vi "Read Registration Refnum.vi"(6 "Event Type":T1, 7 "TreeControlEventHandler":refnum<class "TreeControlEventHandler.lvclass">) -> (1 "TreeControl Refnum":refnum<vi>)   [LabVIEW 2020, in "MVA Framework.lvlib" / "ActorEvents.lvlib" / "TreeControlEventHandler.lvclass"]
doc: "读取注册树形引用"
uses:
  TreeControlEventHandler.lvclass
  <vilib>/event_ctls.llb/lveventtype.ctl
  IEventHandler/IEventHandler.lvclass/IEventHandler.ctl
  TreeControlEventHandler.lvclass/TreeControlEventHandler.ctl
  IEventHandler/IEventHandler.lvclass
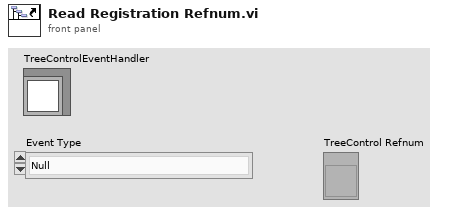
[diagram p1: front panel]
types:
  T1 = typedef "lveventtype.ctl" = enum32{"Null", "Timeout", "Annotation Menu Selection", "Annotation Menu Selection?", "App Instance Close", "App Instance Close?", "Autoscale Range Change", "Bookmark Info Change", "Cell Edit", "Cell Edit?", "Cursor Grab", "Cursor Grab?", "Cursor Menu Selection", "Cursor Menu Selection?", "Cursor Move", "Cursor Release", "Data Change", "Direction Change", "Display State Change", "Drag Ended", "Drag Enter", "Drag Leave", "Drag Over", "Drag Source Update", "Drag Starting", "Drag Starting?", "Drop", "Exec State Change", "Key Down", "Key Down?", "Key Repeat", "Key Repeat?", "Key Up", "Listbox Double Click", "Menu Activation?", "Menu Selection (App)", "Menu Selection? (App)", "Menu Selection (User)", "Mouse Down", "Mouse Down?", "Mouse Enter", "Mouse Leave", "Mouse Move", "Mouse Up", "Mouse Wheel", "NI Security User Change (App)", "Pane Size", "Panel Close", "Panel Close?", "Panel Resize", "Plot Attribute Change", "Scale Range Change", "Shortcut Menu Activation?", "Shortcut Menu Selection (App)", "Shortcut Menu Selection? (App)", "Shortcut Menu Selection (User)", "Tree Double Click", "Tree Drag", "Tree Drag?", "Tree Drop", "Tree Drop?", "Tree Item Close", "Tree Item Close?", "Tree Item Open", "Tree Item Open?", "User Event", "Value Change"}
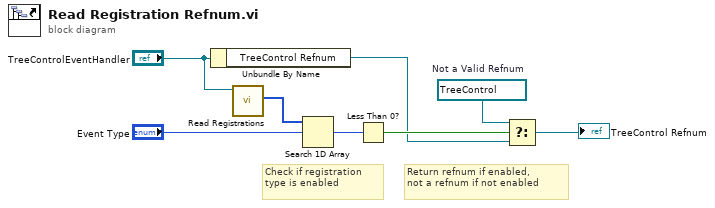
[diagram p0: block diagram]
diagram:
  w1 = refnum<vi> refnum  # Not a Valid Refnum
  # "Return refnum if enabled,\nnot a refnum if not enabled"
  # "Check if registration\ntype is enabled"
  n1 = Unbundle By Name("TreeControlEventHandler") -> ("TreeControl Refnum"=w2:refnum<vi>)
  n2 = call "Read Registrations.vi"("IEventHandler in"="TreeControlEventHandler") -> ("Registrations"=w4:T1[])  [unwired: 10 in]
  n3 = Search 1D Array(1D array=w4, element="Event Type") -> (index of element=w6:i32)  [unwired: 1 in]
  n4 = Less Than 0?(x=w6) -> (x < 0?=w7:bool)
  n5 = Select(t=w1, s=w7, f=w2) -> (s? t:f=→"TreeControl Refnum":refnum<vi>)
